vi "SRS8XX_auto_read.vi"() -> ()   [LabVIEW 2024]
panel:
  out "elapsed time (ms)":u32
  in  "stop":bool
  in  "clear devices\non errors":bool
  out "VISA error?":bool
  out "CH1 and Ch2 output":cluster{"Array":dbl[], "Boolean":bool}[](array[cluster]) {"Array" format="%#_3e"}
  out "Data":dbl[](array[numeric])=[-0.00093841552734, -0.00033187866211, -1.9930615736e-07, -1.0389822336e-09, -0.00070953369141, -0.00042343139648]
  in  "read data?":enum16{"None", "X only", "X Y"}(ring)
  in  "SR 8XX settings":T1(array[cluster])=[{"Instrument Address"="GPIB0::1::INSTR", "parameters"=[0.9, 0.1, 1e-07, 1e-05, 0.0], "channel"=enum."X channel only", "enable"=TRUE, "lockin"=enum."SRS 830"}, {"Instrument Address"="GPIB0::2::INSTR", "parameters"=[0.9, 0.1, 1e-07, 1e-05, 0.0], "channel"=enum."X channel only", "enable"=TRUE, "lockin"=enum."SRS 830"}, {"Instrument Address"="GPIB0::3::INSTR", "parameters"=[0.9, 0.1, 1e-07, 1e-05, 0.0], "channel"=enum."X channel only", "enable"=TRUE, "lockin"=enum."SRS 830"}, {"Instrument Address"="GPIB0::4::INSTR", "parameters"=[0.9, 0.1, 1e-07, 1e-05, 0.0], "channel"=enum."X channel only", "enable"=TRUE, "lockin"=enum."SRS 830"}] {"parameters" format="%.2e"}
  in  "interval between \nreading/sensitivity adjustment (msec)":i32
  # "(works better with read XY data\noption ON)"
  # "Error"
  # "Wiring configuration\n1. Connect CH1 OUT to AUX1 IN\n2. Connect CH2 OUT to AUX2 IN\n3. Set CH1 OUTPUT to X\n4. Set CH2 OUTPUT to Y\n\nThis VI reads the AO of the X and Y channels (10 V for full scale)\nand adjust sensitivity to have the desired sensitivity.\nThe VISA references will be closed every time after execution (slow\nbut seldom interferes with other VI's accessing the lockins). \n\nparameter 0\n  : upper limit for lowering sensitivity\n  ex) 0.9 -> decrease sensitivy when signal\n      reached 90% of the sensitivity\nparameter 1\n   : lower limit for increasing sensitivity\nparameter 2\n     : highest sensitivity\n     sensitivity will not be higher than this value"
  # "highest\nsensitivity(V)"
  # "upper\nlimit"
  # "lower\nlimit"
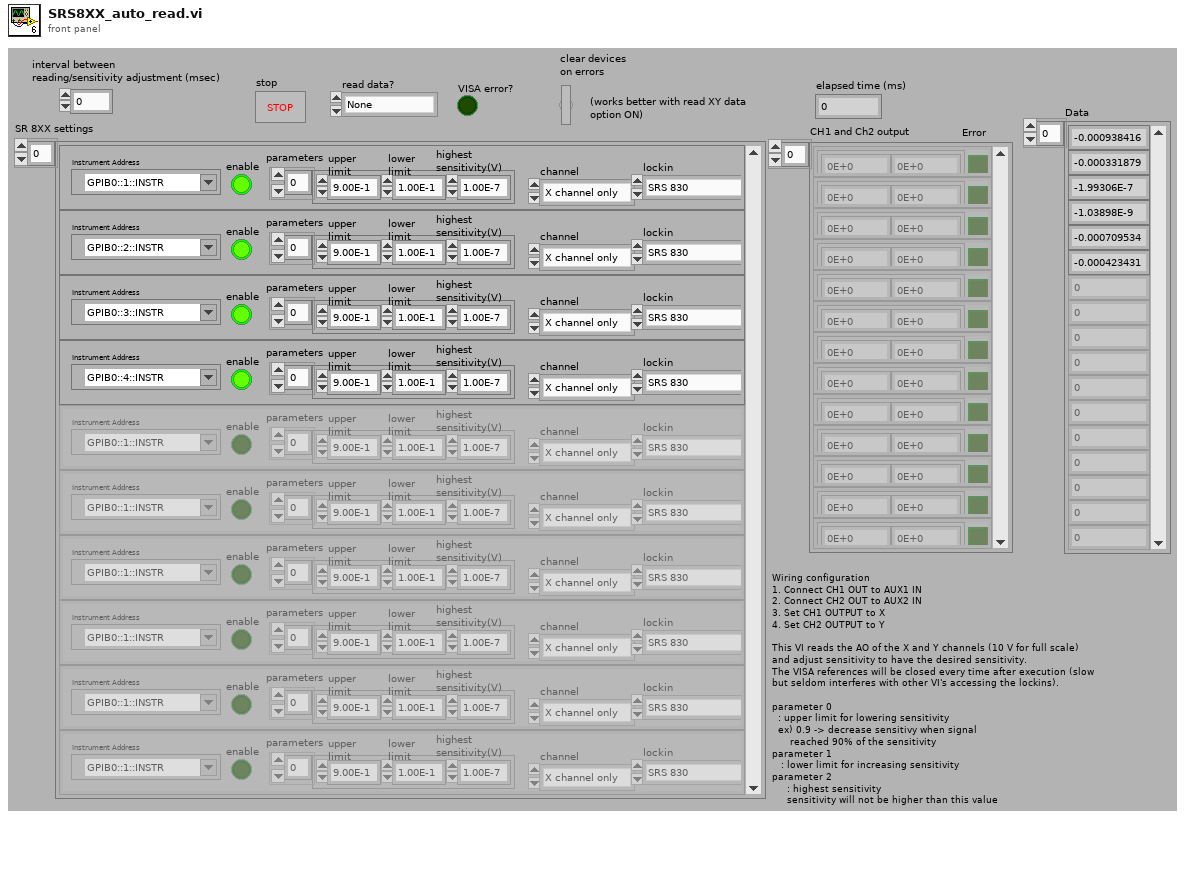
[diagram p1: front panel]
types:
  T1 = cluster{"Instrument Address":refnum<visa-resource-name>, "parameters":dbl[], "channel":enum16{"R ", "X channel only", "Y channel only"}, "enable":bool, "lockin":enum16{"SRS 830", "SRS 86X", "SigRec 72XX"}}[]
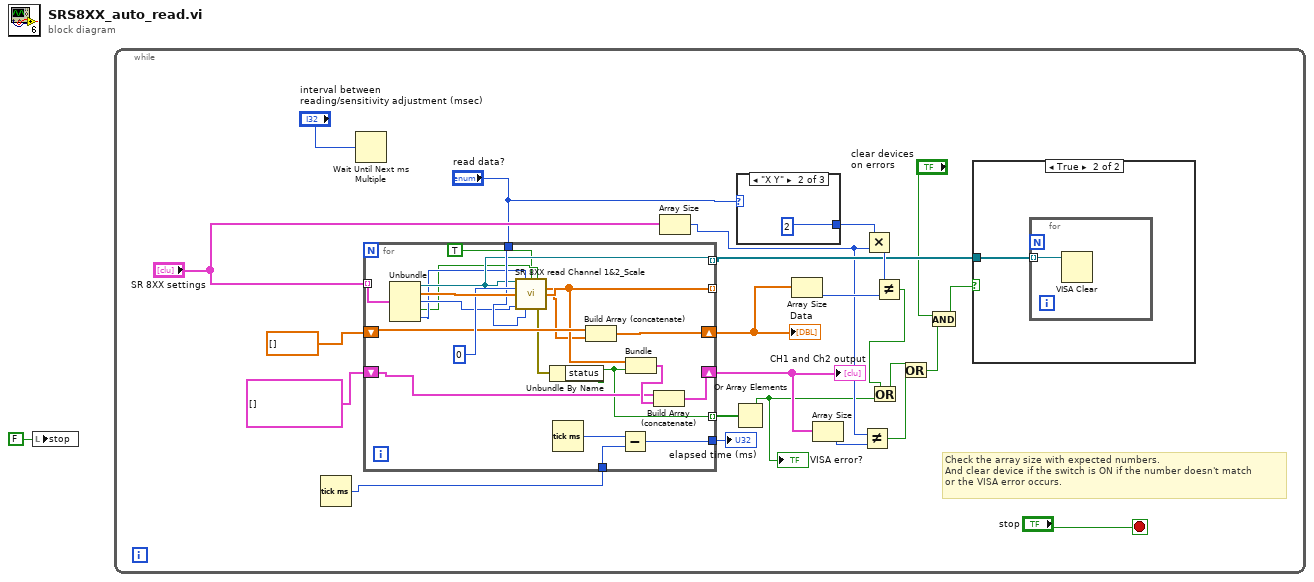
[diagram p0: block diagram]
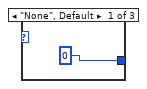
[diagram p3: hidden frame]
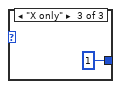
[diagram p4: hidden frame]
diagram:
  n1 = local write "stop"(FALSE ("stop")) -> ()
  n2 = while {
    stop <- "stop" stop-if-true
    # "Check the array size with expected numbers.\nAnd clear device if the switch is ON if the number doesn't match\nor the VISA error occurs."
    n3 = Tick Count (ms)() -> (millisecond timer value=w3:u32)
    n4 = Wait Until Next ms Multiple(millisecond multiple="interval between \nreading/sensitivity adjustment (msec)") -> ()  [unwired: 1 out]
    n5 = for {
      tunnel: "SR 8XX settings" -> [w47] mode=indexing
      tunnel: [w46] -> _ mode=indexing
      shift-right: [w49] -> w17
      shift-left: dbl[] [] -> [w48]
      shift-right: [w43] -> w11
      shift-left: cluster{"CH Output":dbl[], bool}[] [] -> [w42]
      tunnel: [w40] -> w21 mode=indexing
      tunnel: "read data?" -> [w39]
      tunnel: [w38] -> w15 mode=indexing
      tunnel: w3 -> [w36]
      tunnel: [w35] -> w2
      n6 = Unbundle(w47) -> ("Instrument Address"=w38:refnum<visa-resource-name>, "parameters"=w51:dbl[], "channel"=w34:enum16{"R ", "X channel only", "Y channel only"}, "enable"=w32:bool, "lockin"=w33:enum16{"SRS 830", "SRS 86X", "SigRec 72XX"})
      n7 = call "SR 8XX read Channel 1&2_Scale.vi"("Instrument Address"=w38, "lockin"=w33, "close VISA ref."=TRUE, "enable auto?"=w32, "Point #"=0, "parameters_x"=w51, "channel"=w34, "read data"=w39) -> ("Data"=w45:dbl[], "CH Output"=w46:dbl[], "error in (no error) 2"=w41:errorcluster)  [unwired: 2 in, 3 out]
      n8 = Unbundle By Name(w41) -> ("status"=w40:bool)
      n9 = Tick Count (ms)() -> (millisecond timer value=w37:u32)
      n10 = Build Array (concatenate)(w48, w45) -> (w49:dbl[])
      n11 = Subtract(x=w37, y=w36) -> (x-y=w35:u32)
      n12 = Bundle("CH Output"=w46, "status"=w40) -> (w44:cluster{"CH Output":dbl[], "status":bool})  [unwired: 1 in]
      n13 = Build Array (concatenate)(w42, w44) -> (w43:cluster{"CH Output":dbl[], "status":bool}[])
    }
    "Data" <- w17
    "CH1 and Ch2 output" <- w11
    "elapsed time (ms)" <- w2
    n14 = Array Size(array="SR 8XX settings") -> (size(s)=w9:i32)
    n15 = Or Array Elements(Boolean array=w21) -> (logical OR=w7:bool)
    "VISA error?" <- w7
    n16 = case shown="\"X Y\"" "read data?" {
      tunnel: [0 2 1] -> w20
      frame "None", Default {
      }
      frame "X Y" {
      }
      frame "X only" {
      }
    }
    n17 = Array Size(array=w17) -> (size(s)=w19:i32)
    n18 = Array Size(array=w11) -> (size(s)=w10:i32)
    n19 = Not Equal?(x=w9, y=w10) -> (x != y?=w8:bool)
    n20 = Multiply(x=w20, y=w9) -> (x*y=w18:i32)
    n21 = Not Equal?(x=w18, y=w19) -> (x != y?=w13:bool)
    n22 = Or(x=w13, y=w7) -> (x .or. y?=w6:bool)
    n23 = Or(x=w6, y=w8) -> (x .or. y?=w5:bool)
    n24 = And(x="clear devices\non errors", y=w5) -> (x .and. y?=w12:bool)
    n25 = case shown="True" w12 {
      tunnel: w15 -> [_ w26]
      frame False {
      }
      frame True {
        n26 = for {
          tunnel: w26 -> [w27] mode=indexing
          n27 = VISA Clear(VISA resource name=w27) -> ()  [unwired: 1 in, 2 out]
        }
      }
    }
  }
